vi "zlgcan_demo_USBCANFD.vi"() -> ()   [LabVIEW 2021]
doc: "用于设置CAN通道的初始化参数。\n\n适用的设备：USBCANFD-100U、USBCANFD-200U、USBCANFD-MINI"
uses:
  data_type/ZCAN_InitCAN_setting_USBCANFD.ctl
  data_type/ZCAN_Transmit_Data.ctl
  data_type/ZCAN_TransmitFD_Data.ctl
  data_type/CAN Card Type.ctl
  zlgcan.lvlib
panel:
  out "source":string
  in  "开启CAN":bool
  out "CANFD报文显示":string[][](table)
  in  "stop":bool
  in  "?":enum32{"DEMO说明", "设备、通道选择", "参数设置", "状态", "发送"}(tab)
  in  "CAN 通道":u32(ring) items=["0", "1"]
  in  "CAN卡型号":T1=42 items=["USBCANFD-800U"=59, "USBCANFD-200U"=41, "USBCANFD-100U"=42, "USBCANFD-MINI"=43]
  in  "索引":u32(ring) items=["0", "1", "2", "3", "4", "5", "6", "7", "8"]
  in  "仲裁域波特率":u32(ring)=500000 items=["1Mbps"=1000000, "800kbps"=800000, "500kbps"=500000, "250kbps"=250000, "125kbps"=125000, "100kbps"=100000, "50kbps"=50000]
  in  "数据域波特率":u32(ring)=500000 items=["5Mbps"=5000000, "4Mbps"=4000000, "2Mbps"=2000000, "1Mbps"=1000000, "800kbps"=800000, "500kbps"=500000, "250kbps"=250000, "125kbps"=125000, "100kbps"=100000]
  in  "自定义波特率字符输入":string
  in  "自定义波特率开关":bool
  in  "工作模式":u8(ring) items=["正常", "只听"]
  in  "是否使用电阻":u8(ring)=1 items=["不使用终端电阻", "使用终端电阻"]
  out "error out":errorcluster caption="错误输出"
  out "can_index_handle(out)":u32
  out "Device_handle(out)":u32
  in  "帧类型":u32(ring) items=["标准帧", "扩展帧"]
  in  "发送方式":u32(ring) items=["正常发送", "单次发送", "自发自收", "单次自发自收"]
  in  "帧格式":u32(ring) items=["数据帧", "远程帧"]
  out "数据长度":u8=8 max=8
  in  "ID":u32=18 format="0x%08x"
  in  "协议":u32(ring) items=["CAN", "CANFD"]
  in  "数据输入":string="11 22 33 44 55 66 77 88"
  in  "CANFD加速？":u32(ring) items=["不加速", "加速"]
  in  "发送":bool
  in  "CANFD数据帧数组":T2(array[cluster])
  in  "CAN数据帧数组":T3(array[cluster])
  out "CAN报文显示":string[][](table)
  in  "ZCAN_TransmitFD_Data":T4
  in  "ZCAN_Transmit_Data":T5
  in  "ZCAN_InitCAN_Setting_USBCANFD":T6
  out "已接收帧数":u32
  # "适用的设备：USBCANFD-100U、USBCANFD-200U、USBCANFD-MINI、USBCANFD-800U"
  # "停止程序前，\n请先关闭CAN卡"
  # "1. 确保电脑有VC++ 2005/2008/2010/2013运行库（对应32，64位）,微软常用运行库合集，点击下载（35M）。\n    http://manual.zlg.cn/Public/Uploads/2020-06-05/5ed995c271414.zip"
  # "2，如果打开设备失败，可能原因：\n（1）已经打开过一次，没有正常关闭的情况下，继续点击“打开设备”，是无法打开的。\n     需要USB重新拔插，LABVIEW重启（全部关闭），然后再“打开设备”。\n (2) 项目路径不能有中文繁体。"
  # "使用CAN时，\n两个波特率设置相同即可"
  # "使用ZCANPro软件波特率计算工具计算"
  # "CANFD数据长度只能是1~8，12，16，20，24，32，48，64"
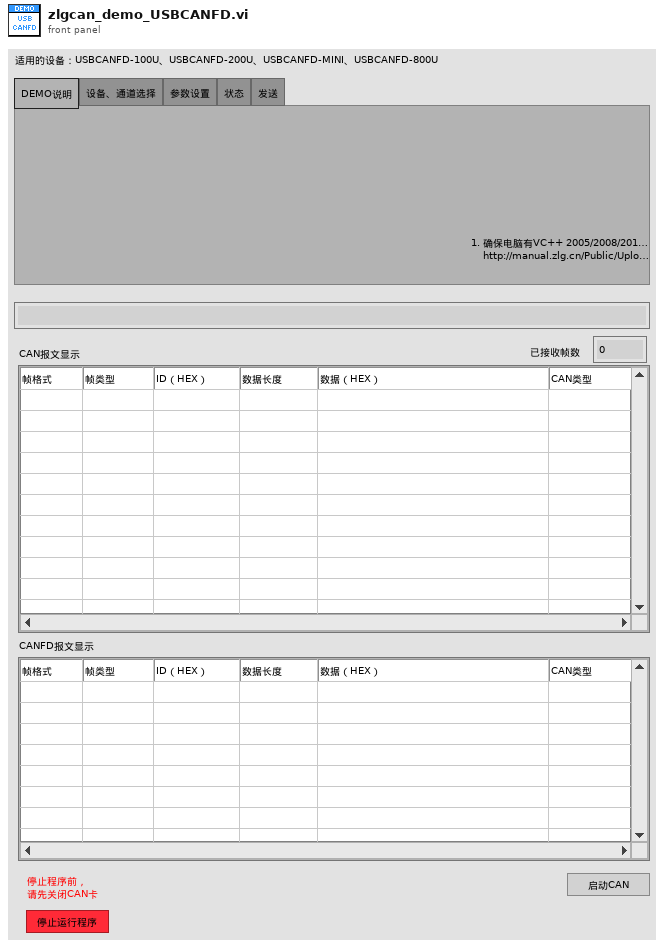
[diagram p1: front panel]
types:
  T1 = typedef "zlgcan.lvlib/CAN Card Type.ctl" = u32
  T2 = cluster{u32, u8, u8, u8, u8, cluster{"[0]":u8, "[1]":u8, "[2]":u8, "[3]":u8, "[4]":u8, "[5]":u8, "[6]":u8, "[7]":u8, "[8]":u8, "[9]":u8, "[10]":u8, "[11]":u8, "[12]":u8, "[13]":u8, "[14]":u8, "[15]":u8, "[16]":u8, "[17]":u8, "[18]":u8, "[19]":u8, "[20]":u8, "[21]":u8, "[22]":u8, "[23]":u8, "[24]":u8, "[25]":u8, "[26]":u8, "[27]":u8, "[28]":u8, "[29]":u8, "[30]":u8, "[31]":u8, "[32]":u8, "[33]":u8, "[34]":u8, "[35]":u8, "[36]":u8, "[37]":u8, "[38]":u8, "[39]":u8, "[40]":u8, "[41]":u8, "[42]":u8, "[43]":u8, "[44]":u8, "[45]":u8, "[46]":u8, "[47]":u8, "[48]":u8, "[49]":u8, "[50]":u8, "[51]":u8, "[52]":u8, "[53]":u8, "[54]":u8, "[55]":u8, "[56]":u8, "[57]":u8, "[58]":u8, "[59]":u8, "[60]":u8, "[61]":u8, "[62]":u8, "[63]":u8}, u64}[]
  T3 = cluster{u32, u8, u8, u8, u8, cluster{"[0]":u8, "[1]":u8, "[2]":u8, "[3]":u8, "[4]":u8, "[5]":u8, "[6]":u8, "[7]":u8}, u64}[]
  T4 = typedef "zlgcan.lvlib/ZCAN_TransmitFD_Data.ctl" = cluster{"帧类型":u32, "帧格式":u32, "ID":u32, "数据长度":u8, "CANFD加速？":u8, "DATA":cluster{"CAN数据[0]":u8, "CAN数据[1]":u8, "CAN数据[2]":u8, "CAN数据[3]":u8, "CAN数据[4]":u8, "CAN数据[5]":u8, "CAN数据[6]":u8, "CAN数据[7]":u8, "CAN数据[8]":u8, "CAN数据[9]":u8, "CAN数据[10]":u8, "CAN数据[11] ":u8, "CAN数据[12] ":u8, "CAN数据[13] ":u8, "CAN数据[14] ":u8, "CAN数据[15] ":u8, "CAN数据[16]":u8, "CAN数据[17]":u8, "CAN数据[18]":u8, "CAN数据[19]":u8, "CAN数据[20]":u8, "CAN数据[21]":u8, "CAN数据[22]":u8, "CAN数据[23]":u8, "CAN数据[24] ":u8, "CAN数据[25]":u8, "CAN数据[26]":u8, "CAN数据[27]":u8, "CAN数据[28]":u8, "CAN数据[29]":u8, "CAN数据[30]":u8, "CAN数据[31]":u8, "CAN数据[32]":u8, "CAN数据[33]":u8, "CAN数据[34]":u8, "CAN数据[35]":u8, "CAN数据[36]":u8, "CAN数据[37]":u8, "CAN数据[38]":u8, "CAN数据[39]":u8, "CAN数据[40]":u8, "CAN数据[41]":u8, "CAN数据[42]":u8, "CAN数据[43]":u8, "CAN数据[44]":u8, "CAN数据[45]":u8, "CAN数据[46]":u8, "CAN数据[47]":u8, "CAN数据[48]":u8, "CAN数据[49]":u8, "CAN数据[50]":u8, "CAN数据[51]":u8, "CAN数据[52]":u8, "CAN数据[53]":u8, "CAN数据[54]":u8, "CAN数据[55]":u8, "CAN数据[56]":u8, "CAN数据[57]":u8, "CAN数据[58]":u8, "CAN数据[59]":u8, "CAN数据[60]":u8, "CAN数据[61]":u8, "CAN数据[62]":u8, "CAN数据[63]":u8}, "发送方式":u32}
  T5 = typedef "zlgcan.lvlib/ZCAN_Transmit_Data.ctl" = cluster{"帧类型":u32, "帧格式":u32, "ID":u32, "数据长度":u8, "DATA":cluster{"CAN数据[0]":u8, "CAN数据[1]":u8, "CAN数据[2]":u8, "CAN数据[3]":u8, "CAN数据[4]":u8, "CAN数据[5]":u8, "CAN数据[6]":u8, "CAN数据[7]":u8}, "发送方式":u32}
  T6 = typedef "zlgcan.lvlib/ZCAN_InitCAN_setting_USBCANFD.ctl" = cluster{"abitbaud":u32, "dbitbaud":u32, "baud_rate_custom？":bool, "RateCustom":string, "mode":u8}
  T7 = cluster{"[0]":u32, "[1]":u32, "[2]":u32, "[3]":u32, "[4]":u32, "[5]":u32, "[6]":u32, "[7]":u32, "[8]":u32, "[9]":u32, "[10]":u32, "[11]":u32, "[12]":u32, "[13]":u32, "[14]":u32, "[15]":u32, "[16]":u32, "[17]":u32, "[18]":u32, "[19]":u32, "[20]":u32, "[21]":u32, "[22]":u32, "[23]":u32, "[24]":u32, "[25]":u32, "[26]":u32, "[27]":u32, "[28]":u32, "[29]":u32, "[30]":u32, "[31]":u32, "[32]":u32, "[33]":u32, "[34]":u32, "[35]":u32, "[36]":u32, "[37]":u32, "[38]":u32, "[39]":u32, "[40]":u32, "[41]":u32, "[42]":u32, "[43]":u32, "[44]":u32, "[45]":u32, "[46]":u32, "[47]":u32, "[48]":u32, "[49]":u32, "[50]":u32, "[51]":u32, "[52]":u32, "[53]":u32, "[54]":u32, "[55]":u32, "[56]":u32, "[57]":u32, "[58]":u32, "[59]":u32, "[60]":u32, "[61]":u32, "[62]":u32, "[63]":u32}
  T8 = cluster{"[0]":u32, "[1]":u32, "[2]":u32, "[3]":u32, "[4]":u32, "[5]":u32, "[6]":u32, "[7]":u32}
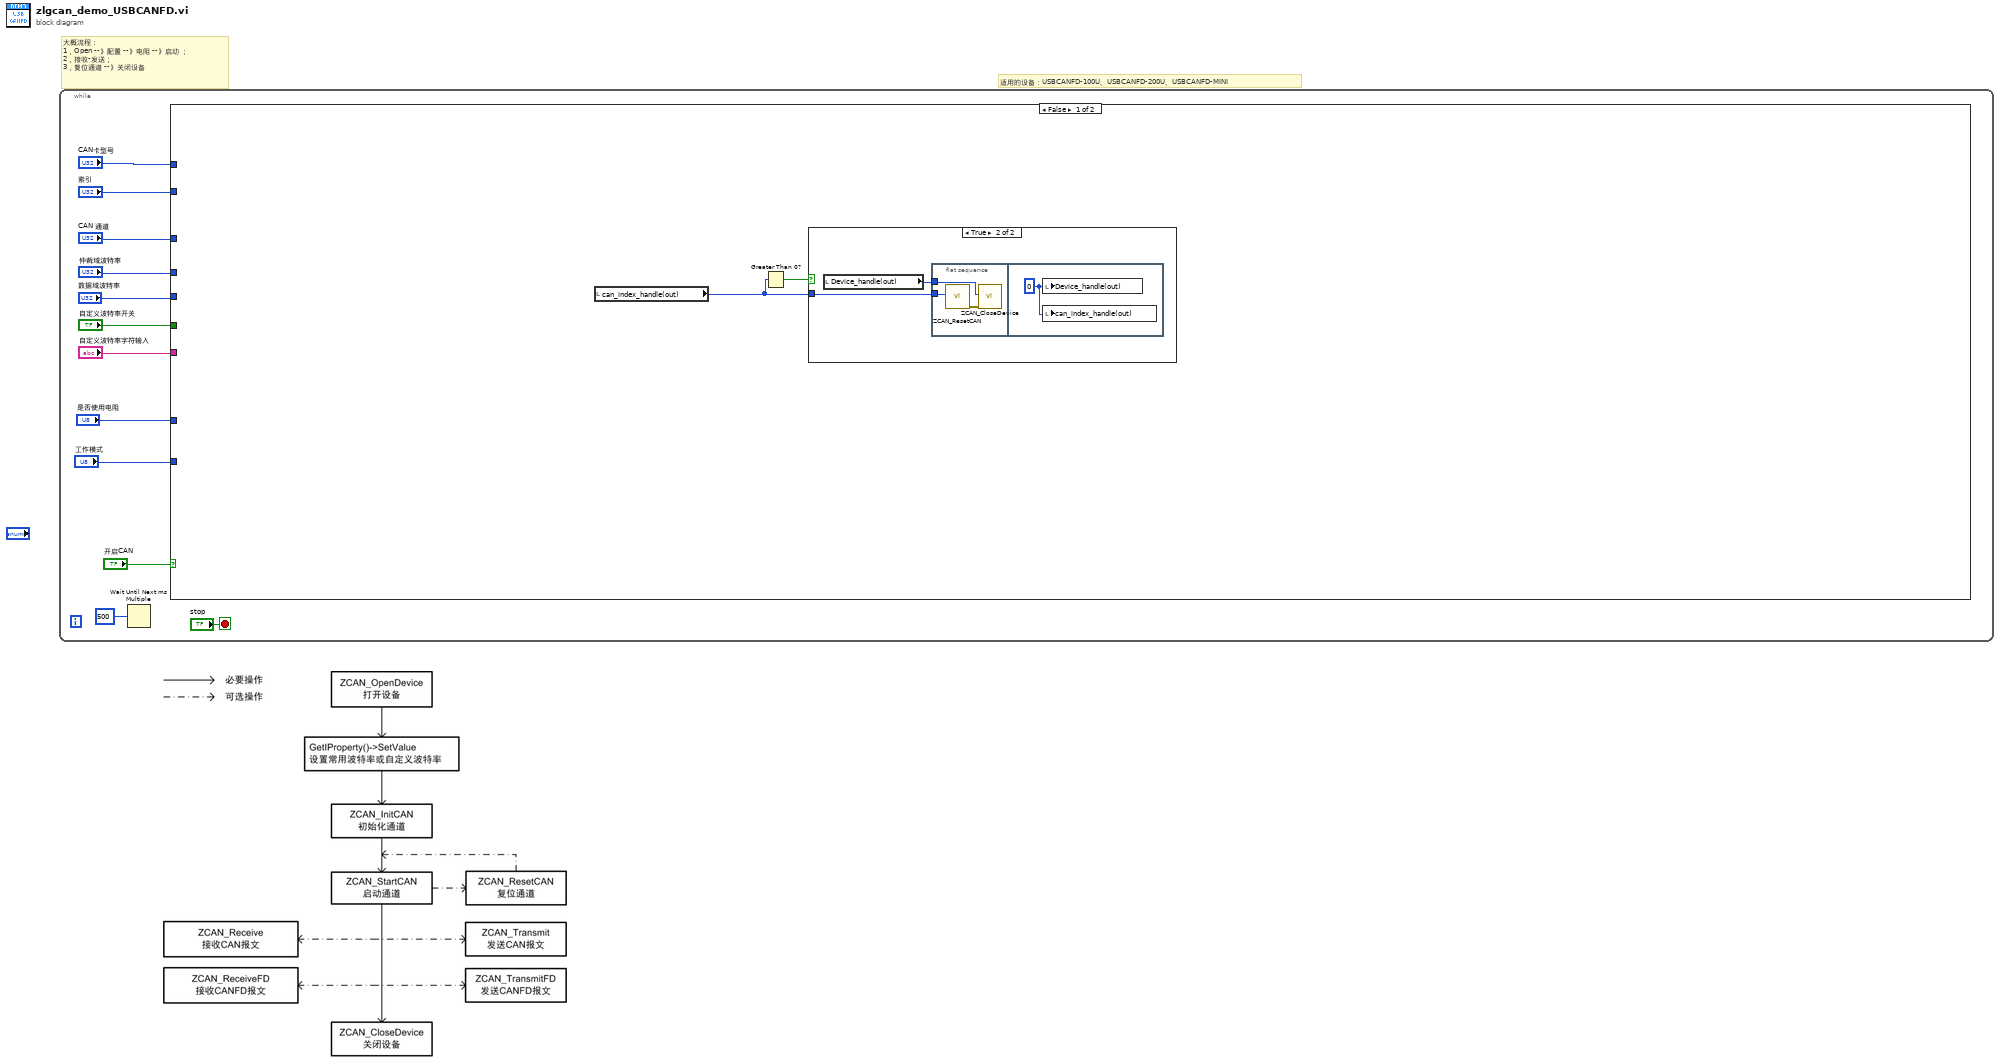
[diagram p0: block diagram]
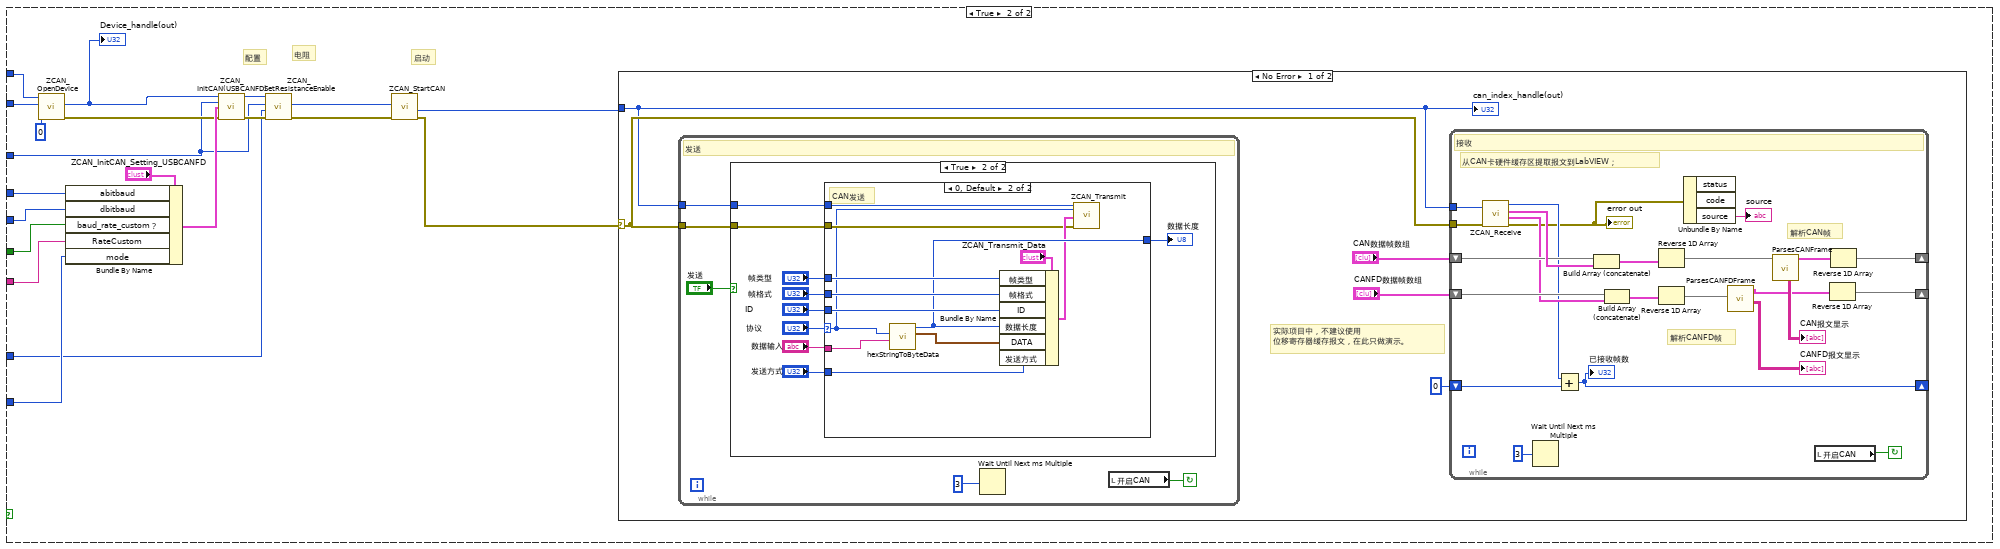
[diagram p3: hidden frame]
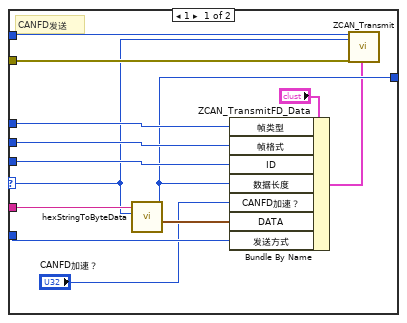
[diagram p5: hidden frame]
diagram:
  # "大概流程：\n1，Open --》配置 --》电阻 --》启动 ；\n2，接收-发送；\n3，复位通道 --》关闭设备"
  # "适用的设备：USBCANFD-100U、USBCANFD-200U、USBCANFD-MINI"
  n1 = while {
    stop <- "stop" stop-if-true
    n2 = Wait Until Next ms Multiple(millisecond multiple=u32 500) -> ()  [unwired: 1 out]
    n3 = case shown="False" "开启CAN" {
      tunnel: "CAN 通道" -> [_ w23]
      tunnel: "仲裁域波特率" -> [_ w33]
      tunnel: "自定义波特率开关" -> [_ w35]
      tunnel: "自定义波特率字符输入" -> [_ w32]
      tunnel: "工作模式" -> [_ w31]
      tunnel: "CAN卡型号" -> [_ w38]
      tunnel: "索引" -> [_ w39]
      tunnel: "数据域波特率" -> [_ w34]
      tunnel: "是否使用电阻" -> [_ w28]
      frame False {
        # "关闭CAN卡"
        n4 = local read "can_index_handle(out)"() -> (w13:u32)
        n5 = Greater Than 0?(x=w13) -> (x > 0?=w14:bool)
        n6 = case shown="True" w14 {
          tunnel: w13 -> [_ w16]
          frame False {
          }
          frame True {
            n7 = local read "Device_handle(out)"() -> (w15:u32)
            n8 = flat-sequence {
              tunnel: w16 -> [w18]
              tunnel: w15 -> [w17]
              frame #0 {
                n9 = call "ZCAN_ResetCAN.vi"("can_handle"=w18) -> ("error out"=w19:errorcluster)  [unwired: 9 in, 1 out]
                n10 = call "ZCAN_CloseDevice.vi"("error in (no error)"=w19, "device_handle"=w17) -> ()  [unwired: 8 in, 2 out]
              }
              frame #1 {
                w20 = u32 0 ("can_index_handle(out)")
                n11 = local write "Device_handle(out)"(w20) -> ()
                n12 = local write "can_index_handle(out)"(w20) -> ()
              }
            }
          }
        }
      }
      frame True {
        # "启动"
        # "电阻"
        # "配置"
        n13 = call "ZCAN_OpenDevice.vi"("reserved"=0, "device_index"=w39, "device_type"=w38) -> ("error out"=w26:errorcluster, "DEVICE_HANDLE"=w24:u32)  [unwired: 7 in]
        "Device_handle(out)" <- w24
        n14 = Bundle By Name(cluster="ZCAN_InitCAN_Setting_USBCANFD", "abitbaud"=w33, "dbitbaud"=w34, "baud_rate_custom？"=w35, "RateCustom"=w32, "mode"=w31) -> (w30:T6)
        n15 = call "ZCAN_InitCAN(USBCANFD).vi"("device_hande"=w24, "can_index"=w23, "ZCAN_InitCAN_Setting_USBCANFD"=w30, "error in (no error)"=w26) -> ("can_index_handle"=w27:u32, "error out"=w29:errorcluster)  [unwired: 10 in]
        n16 = call "ZCAN_SetResistanceEnable.vi"("error in (no error)"=w29, "enable"=w28, "can_index"=w23, "can_index_handle"=w27) -> ("error out"=w22:errorcluster, "can_index_handle(out)"=w25:u32)  [unwired: 6 in]
        n17 = call "ZCAN_StartCAN.vi"("error in (no error)"=w22, "can_index_handle"=w25) -> ("error out"=w21:errorcluster, "can_index_handle(out)"=w37:u32)  [unwired: 7 in, 1 out]
        n18 = case shown="No Error" w21 {
          selector: w21 -> [w44 _]
          tunnel: w37 -> [w43 _]
          frame No Error {
            # "实际项目中，不建议使用\n位移寄存器缓存报文，在此只做演示。"
            n19 = while {
              tunnel: w43 -> [w71]
              tunnel: w44 -> [w69]
              stop <- w70 continue-if-true
              # "发送"
              n20 = case shown="True" "发送" {
                tunnel: w71 -> [_ w75]
                tunnel: w69 -> [_ w76]
                frame False {
                }
                frame True {
                  n21 = case shown="0, Default" "协议" {
                    selector: "协议" -> [w83 w96]
                    tunnel: "帧类型" -> [w94 w106]
                    tunnel: "帧格式" -> [w93 w105]
                    tunnel: "ID" -> [w92 w104]
                    tunnel: "发送方式" -> [w91 w102]
                    tunnel: [w87 w101] -> w77
                    tunnel: "数据输入" -> [w89 w100]
                    tunnel: w76 -> [w86 w98]
                    tunnel: w75 -> [w84 w97]
                    frame 1 {
                      # "CANFD发送"
                      n22 = call "hexStringToByteData.vi"("数据输入"=w89, "协议"=w83) -> ("CANFD_data"=w90:T7, "字节数"=w87:i32)  [unwired: 7 in, 1 out]
                      n23 = Bundle By Name(cluster="ZCAN_TransmitFD_Data", "帧类型"=w94, "帧格式"=w93, "ID"=w92, "数据长度"=w87, "CANFD加速？"="CANFD加速？", "DATA"=w90, "发送方式"=w91) -> (w85:T4)
                      n24 = call "ZCAN_Transmit.vi"("can_index_handle"=w84, "协议"=w83, "error in (no error)"=w86, "ZCAN_TransmitFD_Data"=w85) -> ()  [unwired: 15 in, 1 out]
                    }
                    frame 0, Default {
                      # "CAN发送"
                      n25 = call "hexStringToByteData.vi"("数据输入"=w100, "协议"=w96) -> ("CAN_data"=w103:T8, "字节数"=w101:i32)  [unwired: 7 in, 1 out]
                      n26 = Bundle By Name(cluster="ZCAN_Transmit_Data", "帧类型"=w106, "帧格式"=w105, "ID"=w104, "数据长度"=w101, "DATA"=w103, "发送方式"=w102) -> (w99:T5)
                      n27 = call "ZCAN_Transmit.vi"("can_index_handle"=w97, "协议"=w96, "ZCAN_Transmit_Data"=w99, "error in (no error)"=w98) -> ()  [unwired: 15 in, 1 out]
                    }
                  }
                  "数据长度" <- w77
                }
              }
              n28 = Wait Until Next ms Multiple(millisecond multiple=u32 3) -> ()  [unwired: 1 out]
              n29 = local read "开启CAN"() -> (w70:bool)
            }
            n30 = while {
              tunnel: w44 -> [w66]
              tunnel: w43 -> [w65]
              shift-right: [w67] -> _
              shift-left: 0 -> [w52]
              shift-right: [w56] -> _
              shift-left: "CAN数据帧数组" -> [w62]
              shift-right: [w54] -> _
              shift-left: "CANFD数据帧数组" -> [w60]
              stop <- w64 continue-if-true
              # "从CAN卡硬件缓存区提取报文到LabVIEW；"
              # "解析CANFD帧"
              # "解析CAN帧"
              # "接收"
              n31 = call "ZCAN_Receive.vi"("error in (no error)"=w66, "can_handle"=w65) -> ("error out"=w46:errorcluster, "CANFD数据帧数组"=w59:T2, "CAN数据帧数组"=w63:T3, "Receive_Num"=w53:u32)  [unwired: 2 in]
              "error out" <- w46
              n32 = Wait Until Next ms Multiple(millisecond multiple=u32 3) -> ()  [unwired: 1 out]
              n33 = Add(x=w53, y=w52) -> (x+y=w67:u32)
              "已接收帧数" <- w67
              n34 = Build Array (concatenate)(w62, w63) -> (w61:T3)
              n35 = Build Array (concatenate)(w60, w59) -> (w58:T2)
              n36 = Reverse 1D Array(array=w61) -> (reversed array=w55:T3)
              n37 = Reverse 1D Array(array=w58) -> (reversed array=w50:T2)
              n38 = Unbundle By Name(w46) -> ("source"=→"source":string)  [unwired: 2 out]
              n39 = call "ParsesCANFDFrame.vi"("CANFD数据帧数组"=w50) -> ("CANFD报文显示"=→"CANFD报文显示":string[][], "CANFD数据帧数组(out)"=w49:T2)  [unwired: 9 in]
              n40 = call "ParsesCANFrame.vi"("CAN数据帧数组"=w55) -> ("CAN数据帧数组(out)"=w57:T3, "CAN报文显示"=→"CAN报文显示":string[][])  [unwired: 9 in]
              n41 = local read "开启CAN"() -> (w64:bool)
              n42 = Reverse 1D Array(array=w49) -> (reversed array=w54:T2)
              n43 = Reverse 1D Array(array=w57) -> (reversed array=w56:T3)
            }
            "can_index_handle(out)" <- w43
          }
          frame Error {
          }
        }
      }
    }
  }
